vi "Trigger AI Acquisition.vi"() -> ()   [LabVIEW 2010]
doc: "I. Description:\nThis example demonstrates how to acquire a continuous amount of data (Waveform) using the DAQ device's internal clock.\n\nII. Instructions for Running:\n1. Create an analog input voltage channel.\n2. Set the rate for the sample clock. Additionally, define the sample mode to be continuous.\n3. Call the Start VI to start the acquisition.\n4. Read the waveform data in a loop until the user hits the stop button or an error occurs.\nNote: This example reads data from one or more channels and returns an array of data. Use the Index Array function to access an individual channel of data.\n5. Call the Clear Task VI to clear the Task.\n6. Use the popup dialog box to display an error if any.\n\nIV. I/O Connections Overview:\nMake sure your signal input terminal matches the Physical Channel I/O Control. For further connection information, refer to your hardware reference manual."
uses:
  <vilib>/Utility/error.llb/DialogType.ctl
  <vilib>/DAQmx/read.llb/DAQmx Read (Analog 1D Wfm NChan NSamp).vi
  <vilib>/DAQmx/create/channels.llb/DAQmx Create Channel (AI-Voltage-Basic).vi
  <vilib>/DAQmx/configure/timing.llb/DAQmx Timing (Sample Clock).vi
  <vilib>/DAQmx/configure/trigger.llb/DAQmx Start Trigger (Digital Edge).vi
  <vilib>/daqmx/miscellaneous.llb/DAQmx Fill In Error Info.vi
panel:
  in  "edge":i32(ring)=10280 items=["Rising"=10280, "Falling"=10171]
  in  "source":tag="/Dev1/PFI0"
  in  "Samples to Read":i32=1000
  in  "Physical Channel":tag="Dev1/ai1"
  in  "Minimum Value":dbl=-1.0 format="%0.2f"
  in  "Maximum Value":dbl=1.0 format="%0.2f"
  in  "stop":bool
  in  "Sample Rate":dbl=10000.0 caption="Sample Rate (Hz)" format="%0.2f"
  out "Measurement":waveform(dbl)[](graph)=[{"t0"=timestamp(3331320581.565841 s since 1904-01-01), "dt"=9.999999999999999e-05, "Y"=array[1000 elements], "attributes"=variant("NI_ChannelName"=variant(string "Dev1/ai0"), "NI_UnitDescription"=variant(string "Volts"))}]
  # "For instructions, select Help>>Show Context Help"
  # "Channel Parameters"
  # "Timing Parameters"
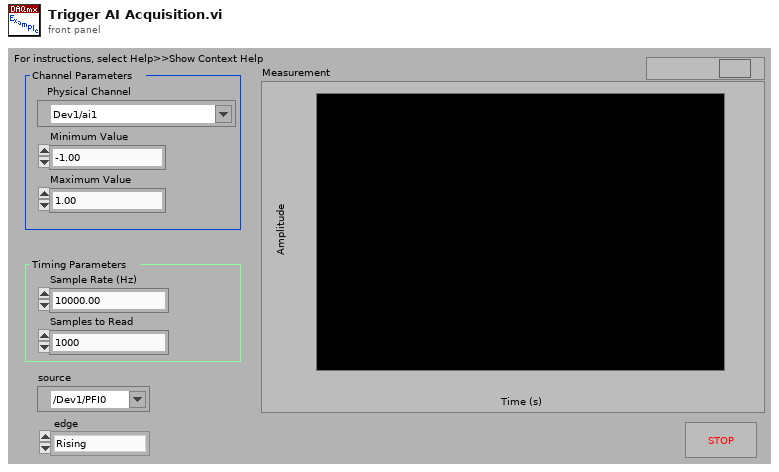
[diagram p1: front panel]
types:
  T1 = typedef "DialogType.ctl" = u16
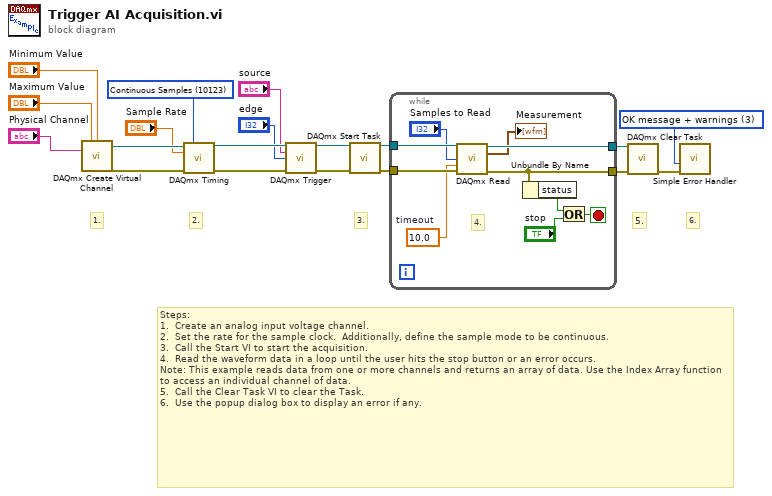
[diagram p0: block diagram]
diagram:
  w7 = T1 3 items=["no dialog", "OK message", "continue or stop message", "OK message + warnings", "continue/stop + warnings"] ("type of dialog (OK msg:1)")
  w10 = 10123 items=["Finite Samples"=10178, "Continuous Samples"=10123] ("sample mode")
  # "6."
  # "5."
  # "Steps: \n1.  Create an analog input voltage channel.\n2.  Set the rate for the sample clock.  Additionally, define the sample mode to be continuous.\n3.  Call the Start VI to start the acquisition.\n4.  Read the waveform data in a loop until the user hits the stop button or an error occurs.\nNote: This example reads data from one or more channels and returns an array of data. Use the Index Array function to access an individual channel of data.\n5.  Call the Clear Task VI to clear the Task.\n6.  Use the popup dialog box to display an error if any."
  # "3."
  # "2."
  # "1."
  n1 = call-poly <vilib>:"DAQmx Create Virtual Channel.vi"("maximum value"="Maximum Value", "minimum value"="Minimum Value", "physical channels"="Physical Channel") -> ("task out"=w14:refnum<k21>, "error out"=w17:errorcluster)  [unwired: 11 in]
  n2 = call-poly <vilib>:"DAQmx Timing.vi"("task/channels in"=w14, "sample mode"=w10, "rate"="Sample Rate", "error in"=w17) -> ("task out"=w3:refnum<k21>, "error out"=w6:errorcluster)  [unwired: 10 in]
  n3 = call-poly <vilib>:"DAQmx Trigger.vi"("task/channels in"=w3, "source"="source", "edge"="edge", "error in"=w6) -> ("task out"=w4:refnum<k21>, "error out"=w5:errorcluster)  [unwired: 10 in]
  n4 = call <vilib>:"DAQmx Start Task.vi"("task/channels in"=w4, "error in"=w5) -> ("task out"=w13:refnum<k21>, "error out"=w16:errorcluster)  [unwired: 12 in]
  n5 = while {
    tunnel: w16 -> [w29]
    tunnel: w13 -> [w28]
    tunnel: [w27] -> w12
    tunnel: [w25] -> w9
    stop <- w23 stop-if-true
    w21 = 10.0  # timeout
    # "4."
    n6 = call-poly <vilib>:"DAQmx Read.vi"("task/channels in"=w28, "number of samples per channel"="Samples to Read", "timeout"=w21, "error in"=w29) -> ("task out"=w27:refnum<k21>, "data"=→"Measurement":waveform(dbl)[], "error out"=w25:errorcluster)  [unwired: 9 in]
    n7 = Unbundle By Name(w25) -> ("status"=w24:bool)
    n8 = Or(x=w24, y="stop") -> (x .or. y?=w23:bool)
  }
  n9 = call <vilib>:"DAQmx Clear Task.vi"("task in"=w12, "error in"=w9) -> ("error out"=w15:errorcluster)  [unwired: 13 in]
  n10 = call <vilib>:"Simple Error Handler.vi"("type of dialog (OK msg:1)"=w7, "error in (no error)"=w15) -> ()  [unwired: 3 in, 5 out]
